vi "单面计算配重2.vi"(0 "vibra_f0":cdb, 1 "vibra_f1":cdb, 3 "错误输入":errorcluster, 7 "f1_weight":dbl, 11 "配重盘孔的数量":dbl, 17 "f1_locate":dbl) -> (10 "err1":dbl, 13 "错误输出":errorcluster, 20 "CW_decomp_f_first_weight":dbl, 21 "CW_decomp_f_first_locate":dbl, 23 "CW_decomp_f_second_weight":dbl, 24 "CW_decomp_f_second_locate":dbl)   [LabVIEW 2014]
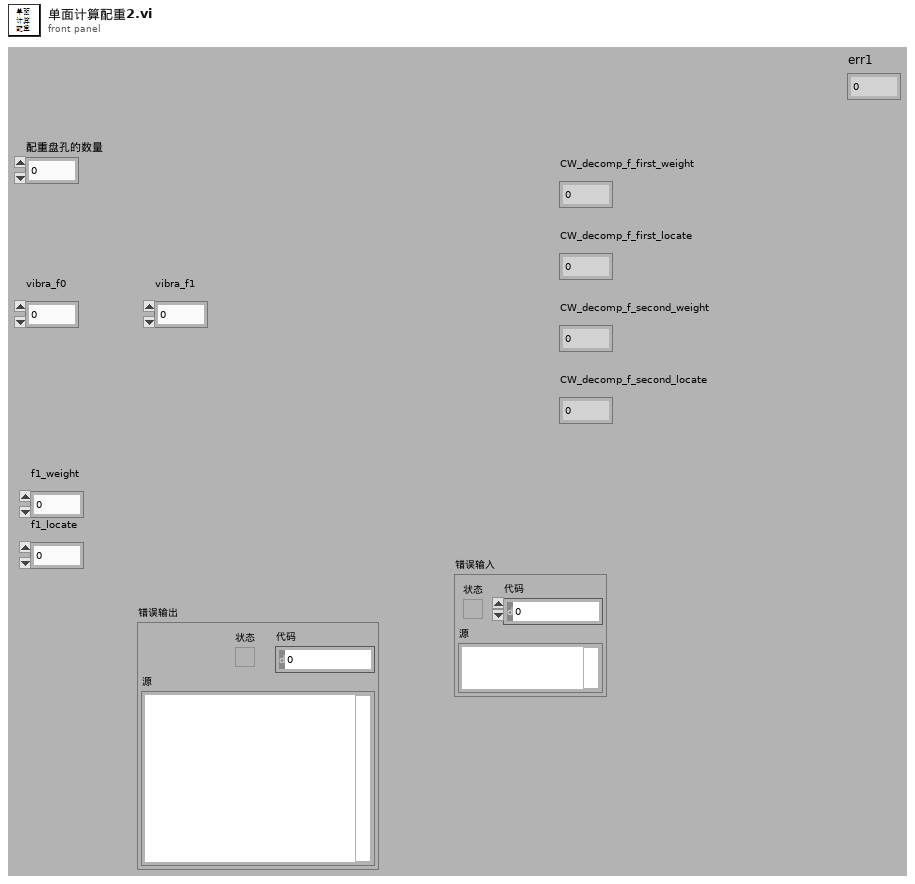
[diagram p1: front panel]
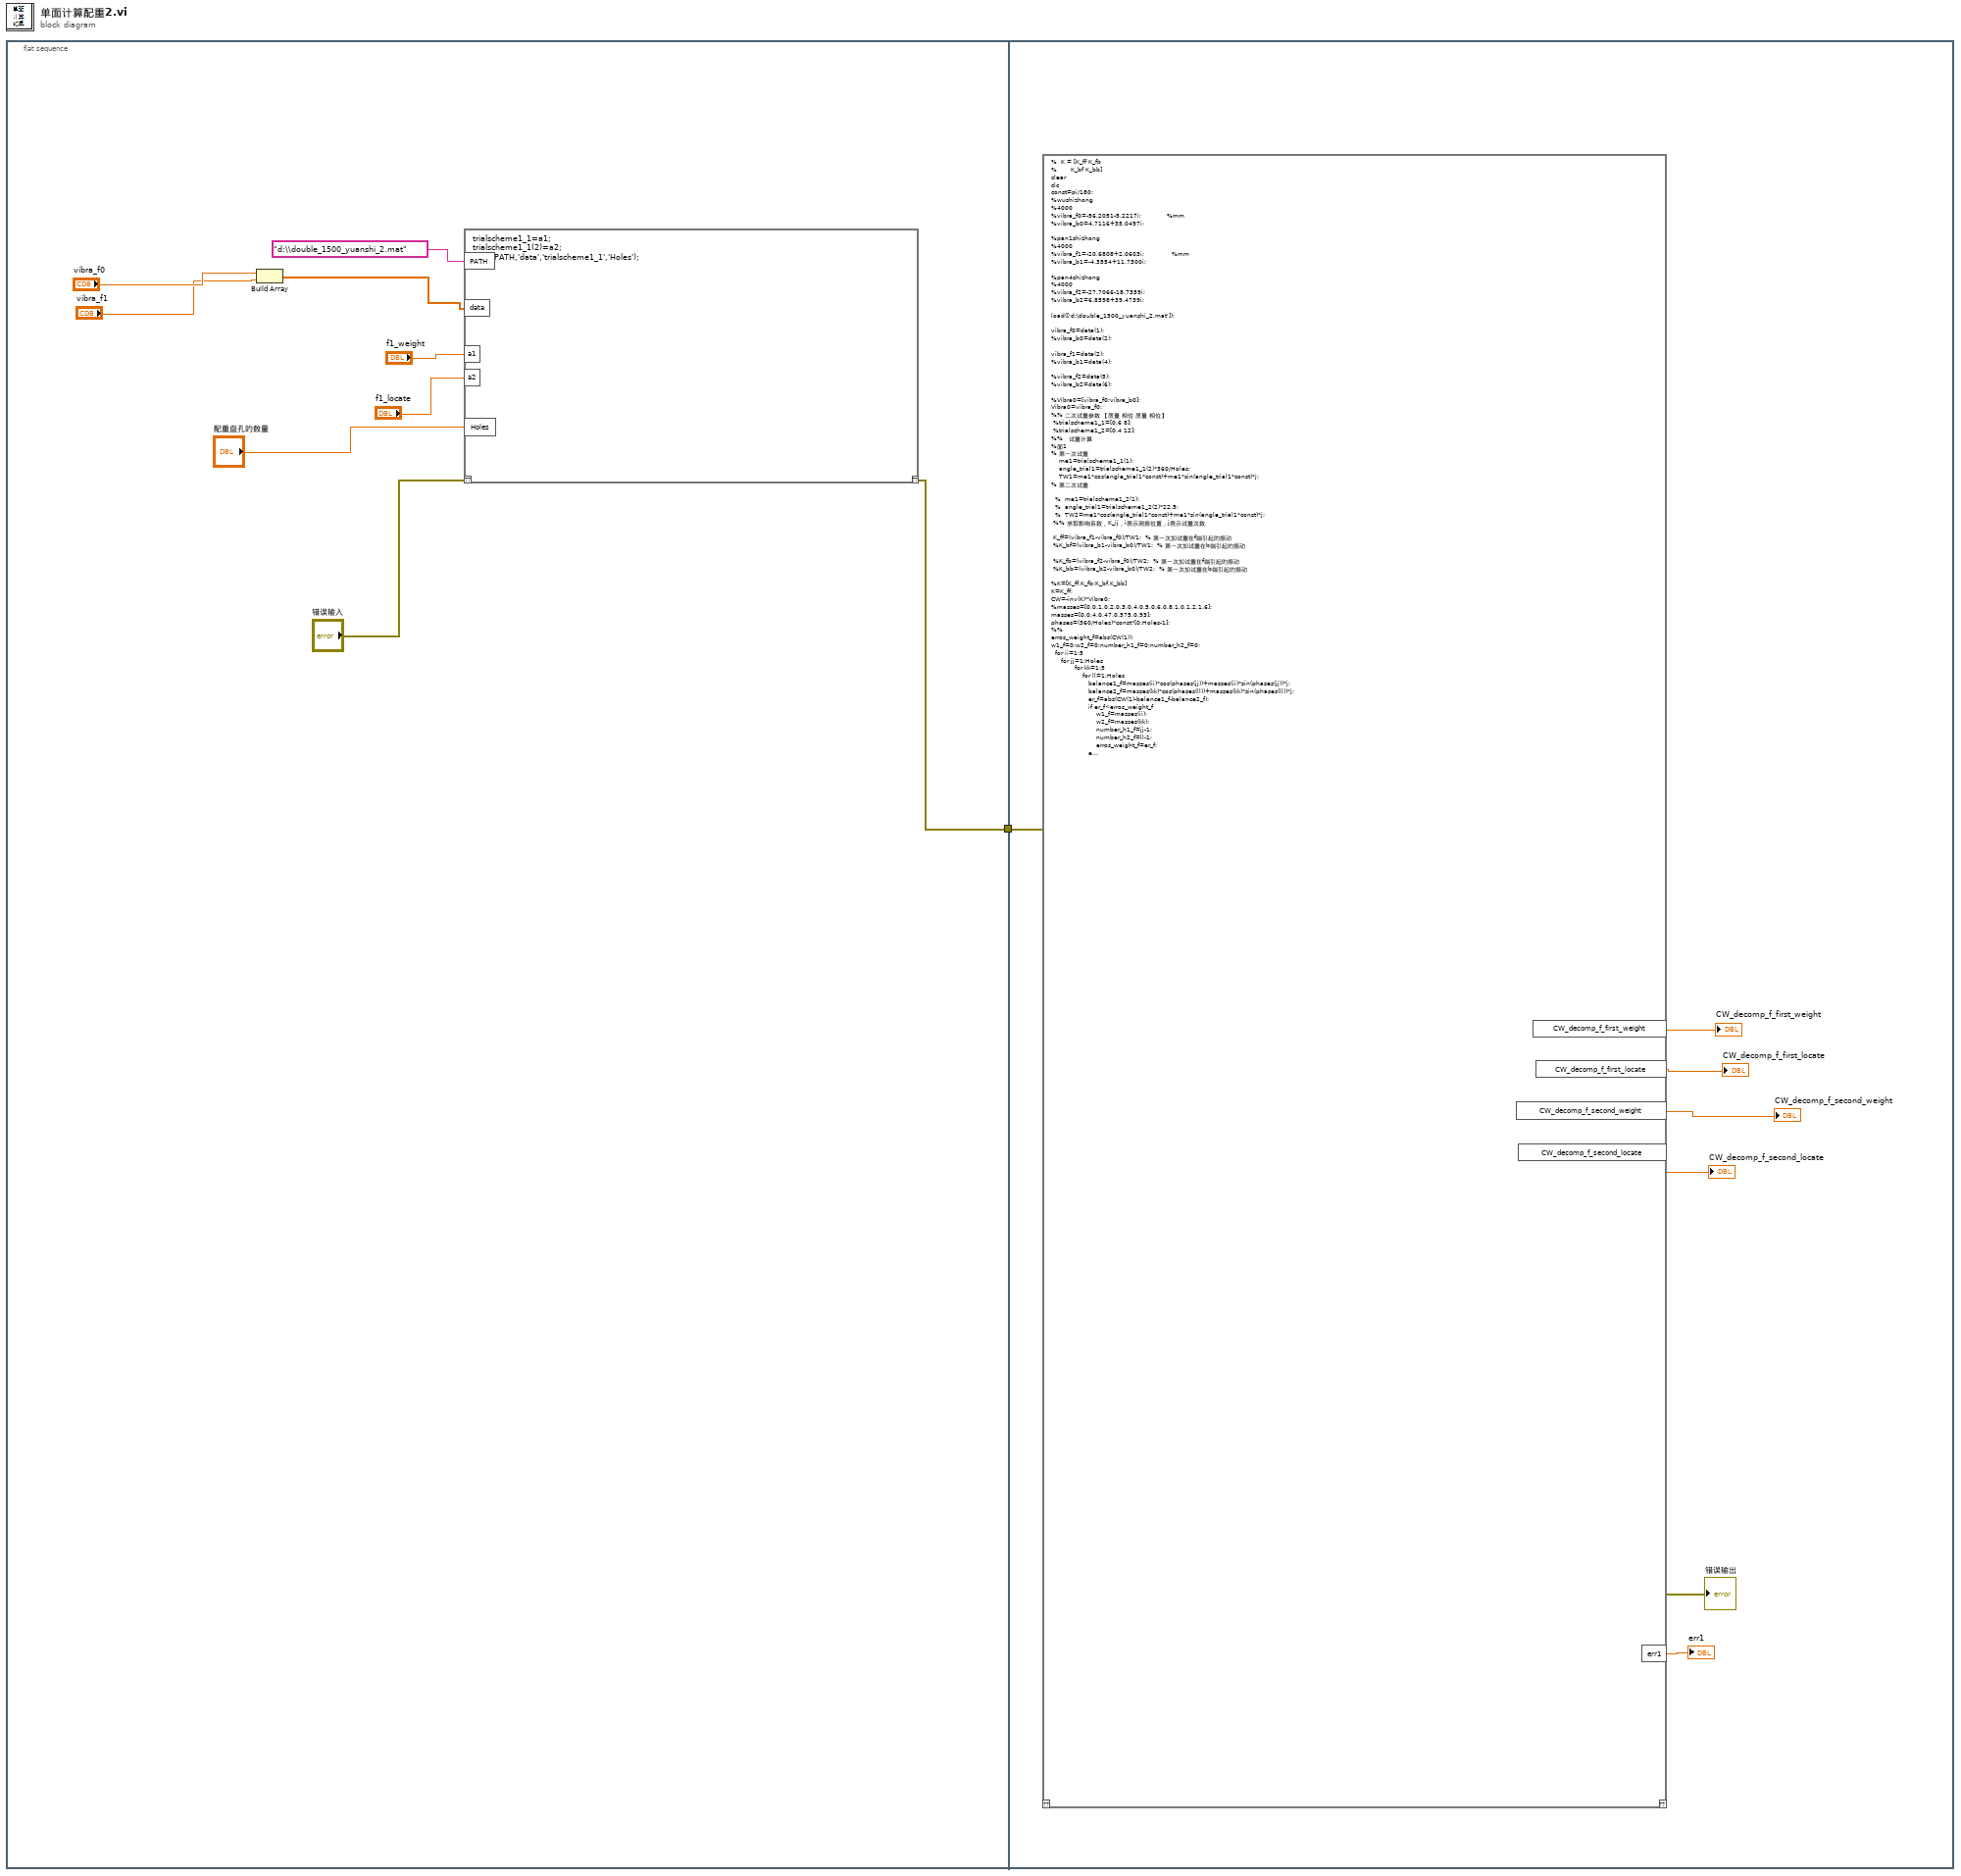
[diagram p0: block diagram]
diagram:
  n1 = flat-sequence {
    tunnel: [w6] -> w1
    tunnel: w1 -> [w17]
    frame #0 {
      n2 = Build Array("vibra_f0", "vibra_f1") -> (w7:cdb[])
      n3 = script code="trialscheme1_1=a1;\ntrialscheme1_1(2)=a2;\nsave(PATH,'data','trialscheme1_1','Holes');"("??"="错误输入", "PATH"="d:\\double_1500_yuanshi_2.mat" ("String"), "data"=w7, "a1"="f1_weight", "a2"="f1_locate", "Holes"="配重盘孔的数量") -> ("??"=w6:errorcluster)
    }
    frame #1 {
      n4 = script code="%  K = [K_ff K_fb\n%       K_bf K_bb]\nclear\nclc\nconst=pi/180;\n%wushizhong\n%4000\n%vibra_f0=-56.2051-5.2217i;             %mm\n%vibra_b0=4.7116+35.0497i;\n\n%pan1shizhong\n%4000\n%vibra_f1=-20.6808+2.0603i;              %mm\n%vibra_b1=-4.3554+11.7300i;\n\n%pan4shizhong\n%4000\n%vibra_f2=-27.7066-18.7359i;\n%vibra_b2=6.8598+39.4739i;\n\nload(['d:\\double_1500_yuanshi_2.mat']);\n\nvibra_f0=data(1);\n%vibra_b0=data(2);\n\nvibra_f1=data(2);\n%vibra_b1=data(4);\n\n%vibra_f2=data(5);\n%vibra_b2=data(6);\n\n%Vibra0=[vibra_f0;vibra_b0];\nVibra0=vibra_f0;\n%% 二次试重参数 【质量 相位 质量 相位】\n %trialscheme1_1=[0.6 8];\n %trialscheme1_2=[0.4 12];\n%%   试重计算 \n%面1\n% 第一次试重\n    me1=trialscheme1_1(1);         \n    angle_trial1=trialscheme1_1(2)*360/Holes;\n    TW1=me1*cos(angle_trial1*const)+me1*sin(angle_trial1*const)*j;\n% 第二次试重 \n\n  %  me1=trialscheme1_2(1);         \n  %  angle_trial1=trialscheme1_2(2)*22.5;\n  %  TW2=me1*cos(angle_trial1*const)+me1*sin(angle_trial1*const)*j;\n %% 求取影响系数，K_ij，i表示测振位置，j表示试重次数\n \n K_ff=(vibra_f1-vibra_f0)/TW1;  % 第一次加试重在f端引起的振动\n %K_bf=(vibra_b1-vibra_b0)/TW1;  % 第一次加试重在b端引起的振动\n\n %K_fb=(vibra_f2-vibra_f0)/TW2;  % 第一次加试重在f端引起的振动\n %K_bb=(vibra_b2-vibra_b0)/TW2;  % 第一次加试重在b端引起的振动\n\n%K=[K_ff,K_fb;K_bf,K_bb]\nK=K_ff;\nCW=-inv(K)*Vibra0;\n%masses=[0,0.1,0.2,0.3,0.4,0.5,0.6,0.8,1.0,1.2,1.6];\nmasses=[0,0.4,0.47,0.575,0.93];\nphases=(360/Holes)*const*[0:Holes-1];\n%%\nerros_weight_f=abs(CW(1));\nw1_f=0;w2_f=0;number_h1_f=0;number_h2_f=0;\n  for ii=1:5\n     for jj=1:Holes\n            for kk=1:5\n                for ll=1:Holes\n                   balance1_f=masses(ii)*cos(phases(jj))+masses(ii)*sin(phases(jj))*j;\n                   balance2_f=masses(kk)*cos(phases(ll))+masses(kk)*sin(phases(ll))*j;\n                   er_f=abs(CW(1)-balance1_f-balance2_f);\n                   if er_f<erros_weight_f\n                       w1_f=masses(ii);\n                       w2_f=masses(kk);\n                       number_h1_f=jj-1;\n                       number_h2_f=ll-1;\n                       erros_weight_f=er_f;\n                   elseif er_f==erros_weight_f&w1_f+w2_f>masses(ii)+masses(kk)\n                          w1_f=masses(ii);\n                          w2_f=masses(kk);\n                          number_h1_f=jj-1;\n                          number_h2_f=ll-1;\n                          erros_weight_f=er_f;\n                          \n                    end\n                end\n            end\n     end\n  end\n balance_scheme_f=[w1_f number_h1_f w2_f number_h2_f erros_weight_f]; \n CW_decomp_f=balance_scheme_f\n\n\nCW_decomp_f_first_weight=CW_decomp_f(1);\nCW_decomp_f_first_locate=CW_decomp_f(2);\nCW_decomp_f_second_weight=CW_decomp_f(3);\nCW_decomp_f_second_locate=CW_decomp_f(4);\n\n\n\nerr1=CW_decomp_f(5);"("??"=w17) -> ("??"=→"错误输出":errorcluster, "CW_decomp_f_first_weight"=→"CW_decomp_f_first_weight":dbl, "CW_decomp_f_first_locate"=→"CW_decomp_f_first_locate":dbl, "CW_decomp_f_second_weight"=→"CW_decomp_f_second_weight":dbl, "CW_decomp_f_second_locate"=→"CW_decomp_f_second_locate":dbl, "err1"=→"err1":dbl)
    }
  }
